vi "Serial Read with Timeout.vi"(6 "Error In (no error)":errorcluster, 7 "Bytes to Read":u32=10, 8 "Timeout Limit":dbl=5.0 format="%.2f", 9 "Resource Name":refnum<visa-resource-name>="ASRL1::INSTR") -> (0 "Error Out":errorcluster, 2 "Serial Read":string, 3 "Dup VISA Resource Name":refnum<visa-resource-name>)   [LabVIEW 2011]
doc: "The Serial Read with Timeout VI will read bytes until either the requested number of bytes is received, or until a timeout occurs."
panel:
  # "Select or enter the serial resource."
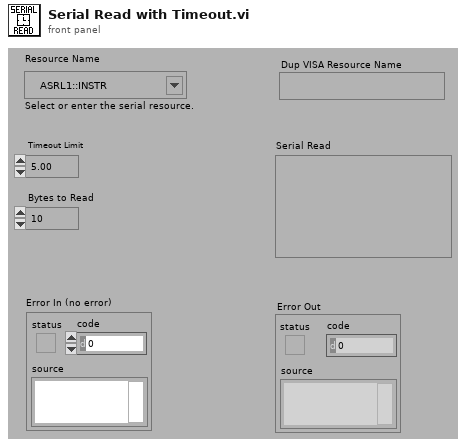
[diagram p1: front panel]
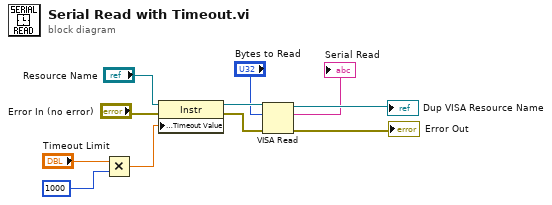
[diagram p0: block diagram]
diagram:
  n1 = Multiply(x="Timeout Limit", y=1000) -> (x*y=w9:dbl)
  n2 = property class="Instr"(reference="Resource Name", error in="Error In (no error)", "General Settings:Timeout Value"=w9) -> (reference out=w7:refnum<visa-resource-name>, error out=w5:errorcluster)
  n3 = VISA Read(VISA resource name=w7, byte count="Bytes to Read", error in (no error)=w5) -> (VISA resource name out=→"Dup VISA Resource Name":refnum<visa-resource-name>, read buffer=→"Serial Read":string, error out=→"Error Out":errorcluster)  [unwired: 1 out]
